vi "作业2（第一题）.vi"() -> ()   [LabVIEW 2017]
panel:
  in  "旋钮":dbl(knob) scale=0.0..10.0
  out "压力表":dbl(knob) scale=0.0..10.0
  out "转速":dbl(knob) scale=0.0..10.0
  out "油表":dbl(slide) scale=0.0..100.0
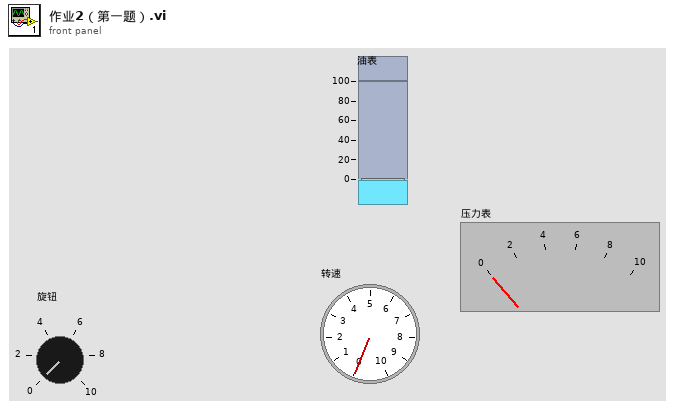
[diagram p1: front panel]
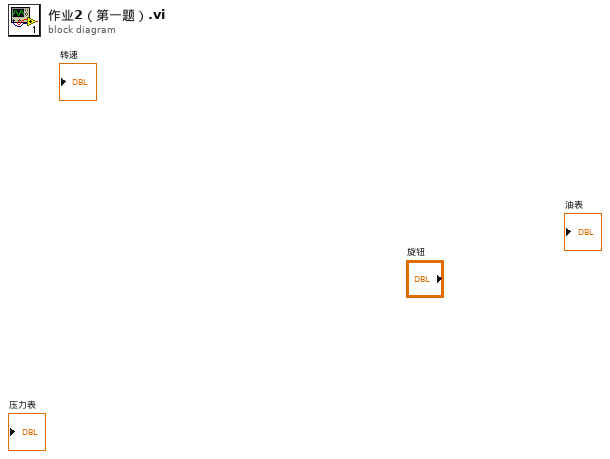
[diagram p0: block diagram]
diagram:
